vi "verify parameters in a list.vi"(8 "error in (no error)":errorcluster, 11 "Simulated_CCD_Camera in":refnum<class "Simulated Camera.lvclass">) -> (0 "error out":errorcluster, 3 "Simulated_CCD_Camera out":refnum<class "Simulated Camera.lvclass">)   [LabVIEW 2018, in "Simulated Camera.lvclass"]
doc: "Verify if the parameters of the camera are in range\n\nThe operating parameters of the CCDs must be within a predefined range. This function verifies if the values provided for these parameters meet this specification. If not, ACS will not allow to start an exposure."
uses:
  Simulated Camera.lvclass
  Simulated Camera.lvclass/Simulated Camera.ctl
panel:
  out "New CCD Config":T1
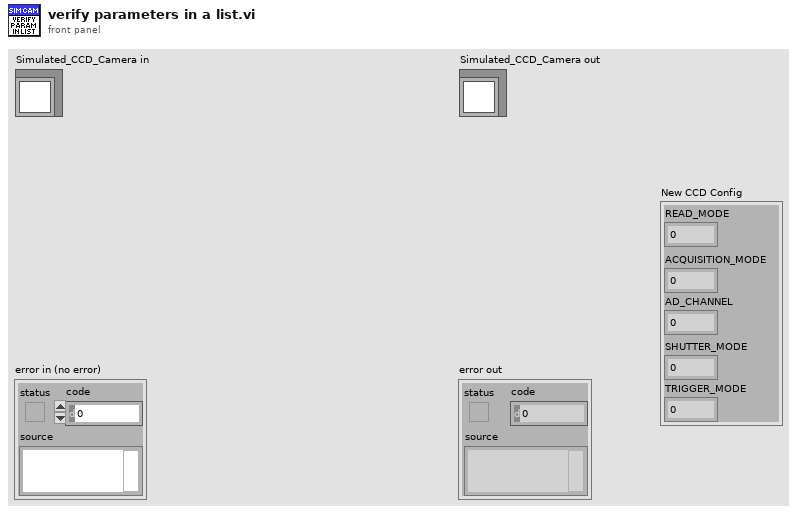
[diagram p1: front panel]
types:
  T1 = cluster{"READ_MODE":u16, "ACQUISITION_MODE":u16, "AD_CHANNEL":u16, "SHUTTER_MODE":u16, "TRIGGER_MODE":u16}
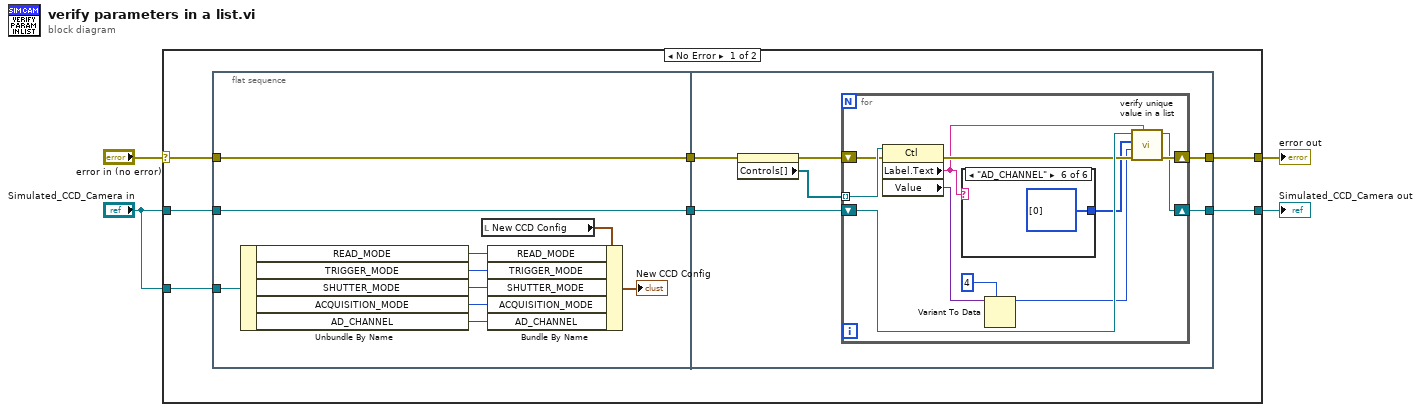
[diagram p0: block diagram]
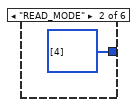
[diagram p3: hidden frame]
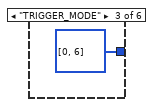
[diagram p4: hidden frame]
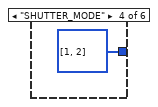
[diagram p5: hidden frame]
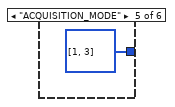
[diagram p6: hidden frame]
diagram:
  n1 = case shown="No Error" "error in (no error)" {
    selector: "error in (no error)" -> [w10 w45]
    tunnel: [w9 w45] -> w3
    tunnel: [w8 w44] -> w2
    tunnel: "Simulated_CCD_Camera in" -> [w11 w44]
    tunnel: "Simulated_CCD_Camera in" -> [w5 _]
    frame No Error {
      n2 = flat-sequence {
        tunnel: w10 -> [w20]
        tunnel: w11 -> [w21]
        tunnel: [w21] -> w7
        tunnel: [w20] -> w6
        tunnel: w5 -> [w12]
        tunnel: [w26] -> w9
        tunnel: [w25] -> w8
        tunnel: w7 -> [w27]
        tunnel: w6 -> [w23]
        frame #0 {
          n3 = Unbundle By Name(w12) -> ("READ_MODE"=w19:u16, "TRIGGER_MODE"=w18:u16, "SHUTTER_MODE"=w17:u16, "ACQUISITION_MODE"=w16:u16, "AD_CHANNEL"=w15:u16)
          n4 = local read "New CCD Config"() -> (w13:T1)
          n5 = Bundle By Name(cluster=w13, "READ_MODE"=w19, "TRIGGER_MODE"=w18, "SHUTTER_MODE"=w17, "ACQUISITION_MODE"=w16, "AD_CHANNEL"=w15) -> (→"New CCD Config":T1)
        }
        frame #1 {
          n6 = property on="New CCD Config" class="Clust (strict)"(error in=w23) -> (error out=w22:errorcluster, "Controls[]"=w24:refnum<vi>[])  [unwired: 1 in, 1 out]
          n7 = for {
            shift-right: [w37] -> w26
            shift-left: w22 -> [w34]
            shift-right: [w36] -> w25
            shift-left: w27 -> [w38]
            tunnel: w24 -> [w35] mode=indexing
            n8 = property class="Ctl"(reference=w35, error in=w34) -> (error out=w33:errorcluster, "Label.Text"=w31:string, "Value"=w30:variant)  [unwired: 1 out]
            n9 = case shown="\"AD_CHANNEL\"" w31 {
              tunnel: [_ i32[] [4] i32[] [0, 6] i32[] [1, 2] i32[] [1, 3] i32[] [0]] -> w32
              frame "False", Default {
              }
              frame "READ_MODE" {
              }
              frame "TRIGGER_MODE" {
              }
              frame "SHUTTER_MODE" {
              }
              frame "ACQUISITION_MODE" {
              }
              frame "AD_CHANNEL" {
              }
            }
            n10 = Variant To Data(type=4, Variant=w30) -> (data=w28:i32)  [unwired: 1 in, 1 out]
            n11 = call "verify unique value in a list.vi"("parameter name"=w31, "error in (no error)"=w33, "value"=w28, "list of values"=w32, "Simulated_CCD_Camera in"=w38) -> ("error out"=w37:errorcluster, "Simulated_CCD_Camera out"=w36:refnum<class "Simulated Camera.lvclass">)  [unwired: 5 in]
          }
        }
      }
    }
    frame Error {
    }
  }
  "error out" <- w3
  "Simulated_CCD_Camera out" <- w2
